vi "Keypad_get_value(SubVI).vi"(0 "Max Value":i32, 5 "I2C Ref  in":T1) -> (7 "Inside array":string, 15 "Output String":string, 17 "Output Array":i32[](array[numeric]), 19 "Number Out":i32)   [LabVIEW 2017]
uses:
  <vilib>/myRIO/Instrument Drivers/Onboard IO/I2C/typedefs/I2C Reference.ctl
  <vilib>/myRIO/Common/Instrument Driver Framework/Utilities/typedefs/myRIO Generic Hardware Reference.ctl
  <vilib>/myRIO/Common/Instrument Driver Framework/Utilities/typedefs/Hardware Version Enum.ctl
  <vilib>/myRIO/Common/Instrument Driver Framework/Utilities/typedefs/myRIO v1.0 Reference.ctl
  <vilib>/myRIO/Common/Instrument Driver Framework/Utilities/typedefs/Generic FPGA Reference.ctl
  <vilib>/myRIO/Common/Instrument Driver Framework/myRIO v1.0/I2C/typedefs/I2C Channels Enum.ctl
  <vilib>/myRIO/Instrument Drivers/Onboard IO/I2C/typedefs/I2C Configuration.ctl
  <vilib>/myRIO/Instrument Drivers/Onboard IO/I2C/typedefs/I2C Transfer Rate.ctl
  <vilib>/myRIO/Instrument Drivers/Onboard IO/DIO/typedefs/DIO Reference.ctl
  <vilib>/myRIO/Common/Instrument Driver Framework/myRIO v1.0/DIO/typedefs/DIO Channels List.ctl
  <vilib>/myRIO/Common/Instrument Driver Framework/myRIO v1.0/DIO/typedefs/DIO Channels Enum.ctl
  <vilib>/userdefined/High Color/nirio_resource_hc.ctl
  <vilib>/myRIO/Common/Instrument Driver Framework/Utilities/vis/Is FPGA Ref Available.vi
  <vilib>/myRIO/Common/Instrument Driver Framework/myRIO v1.0/DIO/vis/myRIO v1.1 Open DIO.vi
  <vilib>/myRIO/Instrument Drivers/Onboard IO/DIO/vis/Read.vi
  <vilib>/myRIO/Common/Instrument Driver Framework/Utilities/vis/Validate Channels.vi
  <vilib>/myRIO/Common/Instrument Driver Framework/myRIO v1.0/DIO/vis/myRIO v1.0 Reserve DIO.vi
  <vilib>/myRIO/Common/Instrument Driver Framework/myRIO v1.0/DIO/vis/myRIO v1.0 Close DIO.vi
  <vilib>/myRIO/Common/Instrument Driver Framework/myRIO v1.0/Resource Manager/vis/myRIO v1.0 Reserve Channel List.vi
  <vilib>/myRIO/Common/Instrument Driver Framework/myRIO v1.0/DIO/vis/myRIO v1.0 Build MUX Configuration DIO.vi
  <vilib>/myRIO/Common/Instrument Driver Framework/myRIO v1.0/DIO/vis/myRIO v1.0 Unreserve DIO.vi
  <vilib>/myRIO/Common/Instrument Driver Framework/myRIO v1.0/Resource Manager/vis/myRIO v1.0 Reserve Channel.vi
  <vilib>/myRIO/Common/Instrument Driver Framework/myRIO v1.0/Resource Manager/vis/myRIO v1.0 Unreserve Channel.vi
  <vilib>/myRIO/Common/Instrument Driver Framework/myRIO v1.0/Resource Manager/vis/myRIO v1.0 Create Configuration List.vi
  <vilib>/myRIO/Common/Instrument Driver Framework/myRIO v1.0/Resource Manager/vis/myRIO v1.0 Unreserve Channel List.vi
  <vilib>/myRIO/Common/Instrument Driver Framework/myRIO v1.0/Resource Manager/vis/myRIO v1.0 Build Mutex Name.vi
  <vilib>/Utility/VariantDataType/GetNumericInfo.vi
  <vilib>/Utility/error.llb/Error Cluster From Error Code.vi
  <vilib>/myRIO/Common/Instrument Driver Framework/myRIO v1.0/myRIO v1.1 Open.vi
  <vilib>/myRIO/Common/Instrument Driver Framework/Utilities/vis/IO Manager.vi
  <vilib>/myRIO/Common/Instrument Driver Framework/Utilities/vis/Configuration Manager.vi
  <vilib>/myRIO/Common/Instrument Driver Framework/myRIO v1.0/Resource Manager/vis/myRIO v1.0 Configure IO.vi
  <vilib>/myRIO/Common/Instrument Driver Framework/myRIO v1.0/myRIO v1.0 Close.vi
  <vilib>/myRIO/Common/Instrument Driver Framework/myRIO v1.0/DIO/vis/myRIO v1.0 Read DIO.vi
  <vilib>/myRIO/Common/Instrument Driver Framework/myRIO v1.0/DIO/vis/myRIO v1.0 Shutdown DIO.vi
  <vilib>/myRIO/Express VI/Onboard IO/DI/DI Express VI.xnode
  <vilib>/myRIO/Instrument Drivers/Onboard IO/DIO/vis/myRIO DIO Open.xnode
  <vilib>/myRIO/Instrument Drivers/Onboard IO/DIO/DIO.lvlib
  <vilib>/myRIO/Instrument Drivers/Onboard IO/I2C/I2C.lvlib
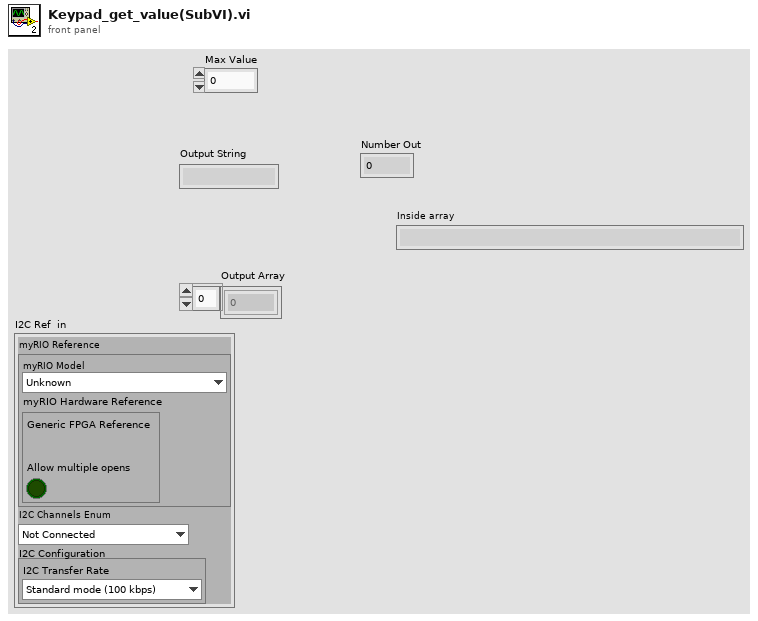
[diagram p1: front panel]
types:
  T1 = typedef "I2C.lvlib/I2C Reference.ctl" = cluster{"myRIO Reference":T2, "I2C Channels Enum":T6, "I2C Configuration":T7}
  T2 = typedef "myRIO Generic Hardware Reference.ctl" = cluster{"myRIO Model":T3, "myRIO Hardware Reference":T4}
  T3 = typedef "Hardware Version Enum.ctl" = enum16{"Unknown", "myRIO-1900", "myRIO-1950", "roboRIO", "NI ELVIS RIO CM"}
  T4 = typedef "myRIO v1.0 Reference.ctl" = cluster{"Generic FPGA Reference":T5, "Allow multiple opens":bool}
  T5 = typedef "Generic FPGA Reference.ctl" = refnum<k20>
  T6 = typedef "I2C Channels Enum.ctl" = enum16{"Not Connected", "A/I2C", "B/I2C", "I2C/I2C"}
  T7 = typedef "I2C.lvlib/I2C Configuration.ctl" = cluster{"I2C Transfer Rate":T8}
  T8 = typedef "I2C.lvlib/I2C Transfer Rate.ctl" = enum16{"Standard mode (100 kbps)", "Fast mode (400 kbps)"}
  T9 = typedef "DIO.lvlib/DIO Reference.ctl" = cluster{"myRIO Reference":T2, "DIO Channels List":T10}
  T10 = typedef "DIO Channels List.ctl" = T11[]
  T11 = typedef "DIO Channels Enum.ctl" = enum16{"Not Connected", "C/DIO0", "C/DIO1", "C/DIO2", "C/DIO3", "C/DIO4", "C/DIO5", "C/DIO6", "C/DIO7", "A/DIO0", "A/DIO1", "A/DIO2", "A/DIO3", "A/DIO4", "A/DIO5", "A/DIO6", "A/DIO7", "A/DIO8", "A/DIO9", "A/DIO10", "A/DIO11", "A/DIO12", "A/DIO13", "A/DIO14", "A/DIO15", "B/DIO0", "B/DIO1", "B/DIO2", "B/DIO3", "B/DIO4", "B/DIO5", "B/DIO6", "B/DIO7", "B/DIO8", "B/DIO9", "B/DIO10", "B/DIO11", "B/DIO12", "B/DIO13", "B/DIO14", "B/DIO15", "LED0", "LED1", "LED2", "LED3", "Button0", "DIO/DIO0", "DIO/DIO1", "DIO/DIO2", "DIO/DIO3", "DIO/DIO4", "DIO/DIO5", "DIO/DIO6", "DIO/DIO7", "DIO/DIO8", "DIO/DIO9", "SPI/CS0", "SPI/CS1", "SPI/CS2", "SPI/CS3", "LED RADIO (Green)", "LED RADIO (Red)", "LED COMM (Green)", "LED COMM (Red)", "LED MODE (Green)", "LED MODE (Red)"}
  T12 = typedef "nirio_resource_hc.ctl" = tag
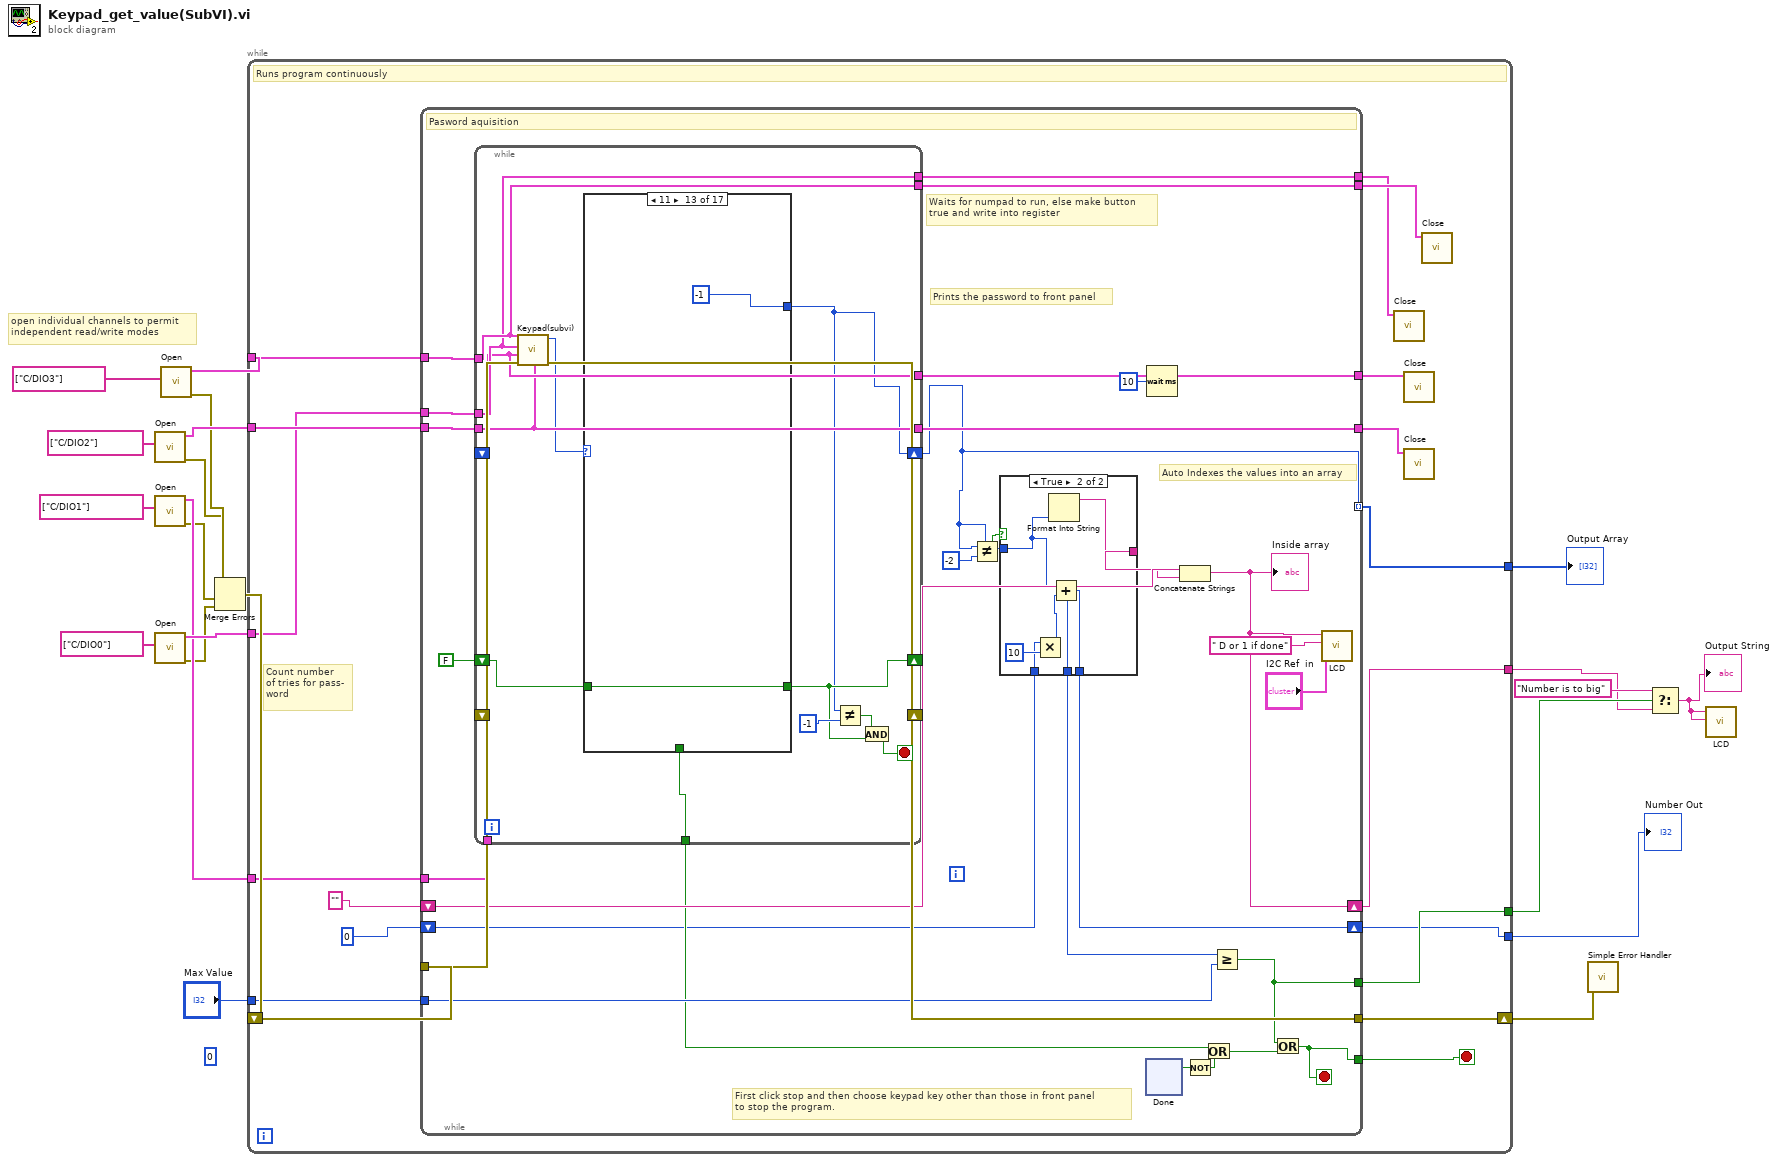
[diagram p0: block diagram]
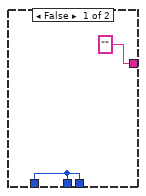
[diagram p2: hidden frame]
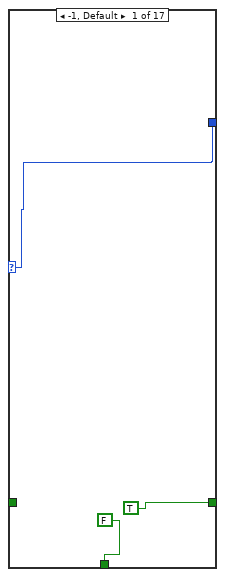
[diagram p3: hidden frame]
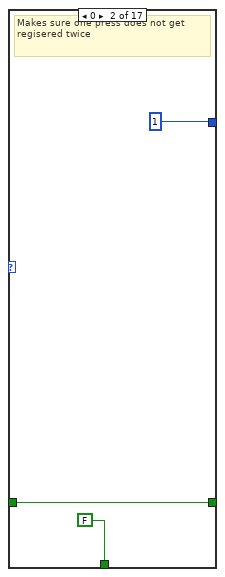
[diagram p4: hidden frame]
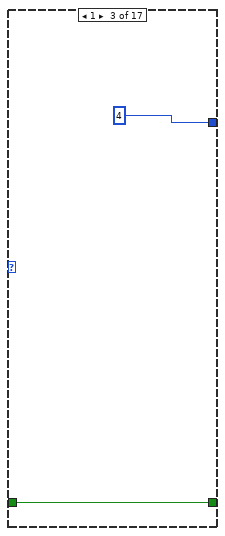
[diagram p5: hidden frame]
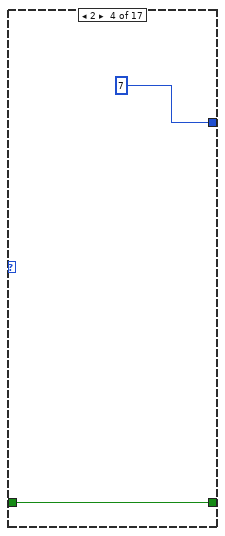
[diagram p6: hidden frame]
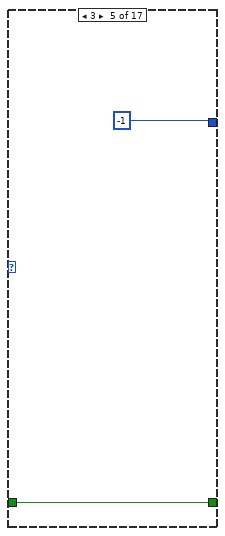
[diagram p7: hidden frame]
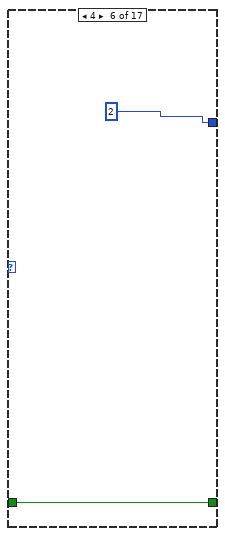
[diagram p8: hidden frame]
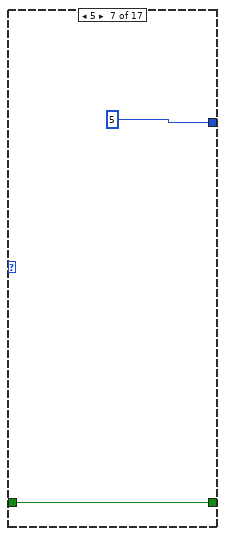
[diagram p9: hidden frame]
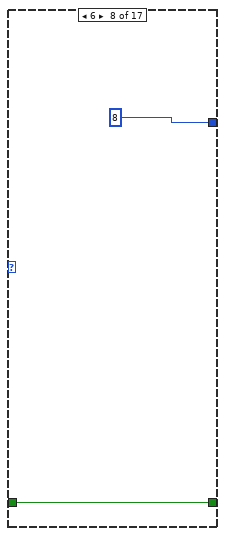
[diagram p10: hidden frame]
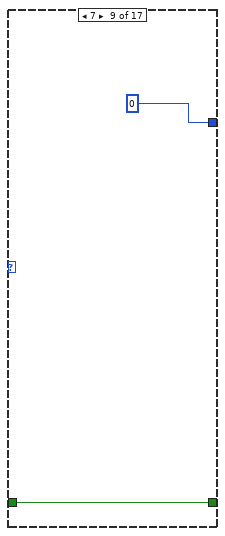
[diagram p11: hidden frame]
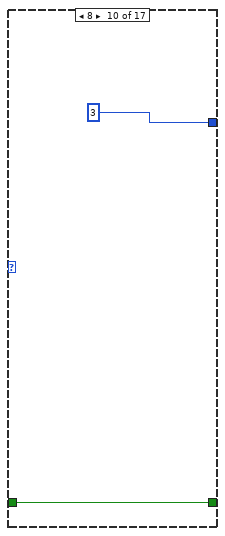
[diagram p12: hidden frame]
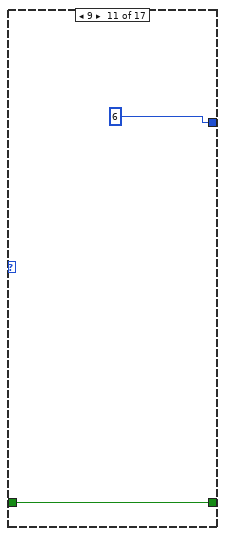
[diagram p13: hidden frame]
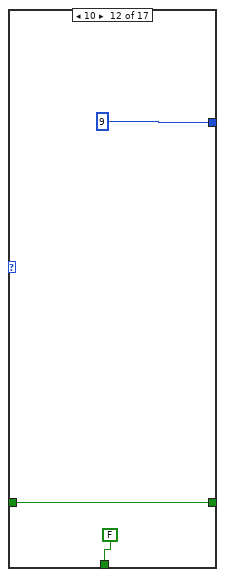
[diagram p14: hidden frame]
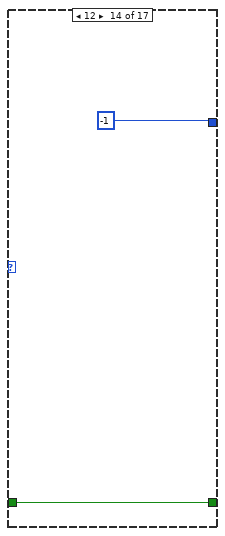
[diagram p15: hidden frame]
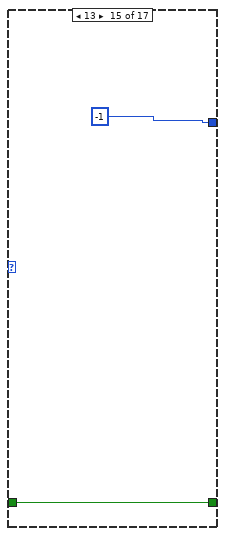
[diagram p16: hidden frame]
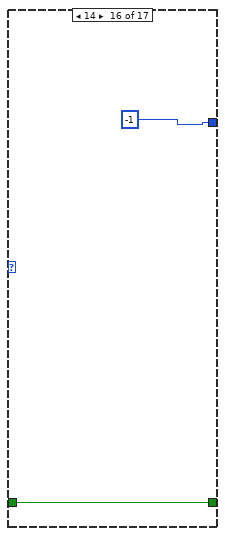
[diagram p17: hidden frame]
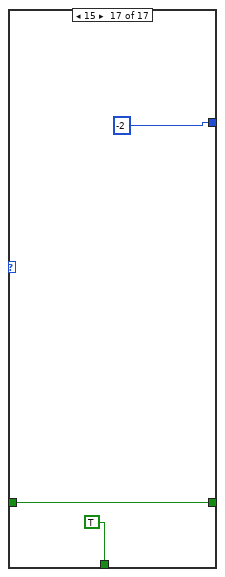
[diagram p18: hidden frame]
diagram:
  (unwired) 0
  # "open individual channels to permit\nindependent read/write modes"
  n1 = call <vilib>:"Open.vi"("Channel Names"=tag[] ["C/DIO2"]) -> ("error out"=w13:errorcluster, "DIO Ref Out"=w16:T9)  [unwired: 9 in]
  n2 = call <vilib>:"Open.vi"("Channel Names"=tag[] ["C/DIO1"]) -> ("error out"=w12:errorcluster, "DIO Ref Out"=w17:T9)  [unwired: 9 in]
  n3 = call <vilib>:"Open.vi"("Channel Names"=tag[] ["C/DIO0"]) -> ("error out"=w11:errorcluster, "DIO Ref Out"=w18:T9)  [unwired: 9 in]
  n4 = call <vilib>:"Open.vi"("Channel Names"=tag[] ["C/DIO3"]) -> ("error out"=w14:errorcluster, "DIO Ref Out"=w15:T9)  [unwired: 9 in]
  n5 = Merge Errors "Merge Errors"(w14, w13, w12, w11) -> (w19:errorcluster)
  n6 = while {
    tunnel: w15 -> [w39]
    tunnel: w16 -> [w38]
    tunnel: w17 -> [w37]
    tunnel: w18 -> [w36]
    shift-right: [w34] -> w20
    shift-left: w19 -> [w35]
    tunnel: [w32] -> w21
    tunnel: [w31] -> w3
    tunnel: "Max Value" -> [w30]
    tunnel: [w28] -> w5
    tunnel: [w23] -> w2
    stop <- w29 stop-if-true
    # "Count number \nof tries for pass-\nword"
    # "Runs program continuously"
    n7 = while {
      tunnel: w39 -> [w68]
      tunnel: w38 -> [w64]
      tunnel: w37 -> [w66]
      tunnel: w36 -> [w65]
      tunnel: w35 -> [w67]
      tunnel: [w63] -> w34
      tunnel: [w44] -> w32 mode=indexing
      shift-right: [w54] -> w31
      shift-left: "" -> [w61]
      tunnel: w30 -> [w57]
      tunnel: [w56] -> w29
      tunnel: [w55] -> w28
      tunnel: [w49] -> w27
      tunnel: [w48] -> w26
      tunnel: [w47] -> w25
      tunnel: [w46] -> w24
      shift-right: [w42] -> w23
      shift-left: 0 -> [w41]
      stop <- w56 stop-if-true
      # "Auto Indexes the values into an array"
      # "Waits for numpad to run, else make button\ntrue and write into register"
      # "Prints the password to front panel"
      # "First click stop and then choose keypad key other than those in front panel \nto stop the program."
      # "Pasword aquisition"
      n8 = while {
        tunnel: w68 -> [w118]
        tunnel: w66 -> [w116]
        tunnel: w65 -> [w117]
        tunnel: w64 -> [w115]
        shift-right: [w125] -> w63
        shift-left: w67 -> [w126]
        shift-right: [w114] -> w44
        shift-left: _ -> [_]
        shift-right: [w121] -> _
        shift-left: FALSE -> [w124]
        tunnel: [w119] -> w52
        tunnel: [w118] -> w49
        tunnel: [w117] -> w48
        tunnel: [w116] -> w47
        tunnel: [w115] -> w46
        stop <- w120 stop-if-true
        n9 = call "Keypad(subvi).vi"("DIO Ref Out 4"=w118, "error in (no error)"=w126, "DIO Ref Out"=w116, "DIO Ref Out 2"=w117, "DIO Ref Out 3"=w115) -> ("error out"=w125:errorcluster, "Index of current pressed button"=w113:i32)  [unwired: 3 in, 2 out]
        n10 = case shown="11" w113 {
          selector: w113 -> [w127 _ _ _ _ _ _ _ _ _ _ _ _ _ _ _ _]
          tunnel: [w127 1 4 7 -1 2 5 8 0 3 6 9 -1 -1 -1 -1 -2] -> w114
          tunnel: [TRUE w132 w134 w136 w138 w140 w142 w144 w146 w148 w150 w153 w155 w157 w159 w161 w164] -> w121
          tunnel: w124 -> [_ w132 w134 w136 w138 w140 w142 w144 w146 w148 w150 w153 w155 w157 w159 w161 w164]
          tunnel: [FALSE FALSE _ _ _ _ _ _ _ _ _ FALSE _ _ _ _ TRUE] -> w119
          frame -1, Default {
          }
          frame 0 {
            # "Makes sure one press does not get regisered twice"
          }
          frame 1 {
          }
          frame 2 {
          }
          frame 3 {
          }
          frame 4 {
          }
          frame 5 {
          }
          frame 6 {
          }
          frame 7 {
          }
          frame 8 {
          }
          frame 9 {
          }
          frame 10 {
          }
          frame 11 {
          }
          frame 12 {
          }
          frame 13 {
          }
          frame 14 {
          }
          frame 15 {
          }
        }
        n11 = Not Equal?(x=w114, y=-1) -> (x != y?=w122:bool)
        n12 = And(x=w122, y=w121) -> (x .and. y?=w120:bool)
      }
      n13 = Not Equal?(x=w44, y=-2) -> (x != y?=w58:bool)
      n14 = case shown="True" w58 {
        tunnel: w44 -> [_ w110]
        tunnel: ["" w112] -> w60
        tunnel: [w105 w111] -> w43
        tunnel: [w105 w111] -> w42
        tunnel: w41 -> [w105 w108]
        frame False {
        }
        frame True {
          n15 = Multiply(x=w108, y=10) -> (x*y=w107:i32)
          n16 = Format Into String(w110) -> (resulting string=w112:string)  [unwired: 3 in, 1 out]
          n17 = Add(x=w110, y=w107) -> (x+y=w111:i32)
        }
      }
      n18 = xnode "Done"() -> ("B/DIO4 (Pin 19)"=w50:bool)  [unwired: 1 in, 1 out]
      n19 = Wait (ms)(milliseconds to wait=u32 10) -> ()  [unwired: 1 out]
      n20 = Concatenate Strings(w61, w60) -> (w54:string)
      "Inside array" <- w54
      n21 = Not(x=w50) -> (.not. x?=w45:bool)
      n22 = Or(x=w52, y=w45) -> (x .or. y?=w51:bool)
      n23 = Greater Or Equal?(x=w43, y=w57) -> (x >= y?=w55:bool)
      n24 = Or(x=w55, y=w51) -> (x .or. y?=w56:bool)
      n25 = call "LCD.vi"("I2C Ref  in"="I2C Ref  in", "String 2"=" D or 1 if done", "String"=w54) -> ()  [unwired: 8 in, 1 out]
    }
    n26 = call <vilib>:"Close.vi"("DIO Ref In"=w26) -> ()  [unwired: 10 in, 1 out]
    n27 = call <vilib>:"Close.vi"("DIO Ref In"=w25) -> ()  [unwired: 10 in, 1 out]
    n28 = call <vilib>:"Close.vi"("DIO Ref In"=w24) -> ()  [unwired: 10 in, 1 out]
    n29 = call <vilib>:"Close.vi"("DIO Ref In"=w27) -> ()  [unwired: 10 in, 1 out]
  }
  "Output Array" <- w21
  "Number Out" <- w2
  n30 = call <vilib>:"Simple Error Handler.vi"("error in (no error)"=w20) -> ()  [unwired: 4 in, 5 out]
  n31 = Select(t="Number is to big", s=w5, f=w3) -> (s? t:f=w1:string)
  "Output String" <- w1
  n32 = call "LCD.vi"("String 2"=w1, "String"=w1) -> ()  [unwired: 9 in, 1 out]
